vi "Smax.vi"(8 "error in ( error)":errorcluster, 10 "Pair Channel":waveform(sgl), 11 "Data":waveform(sgl)) -> (0 "error out":errorcluster, 3 "Smax":sgl)   [LabVIEW 2017, in "VibrationAnalysisFunctions.lvlib"]
uses:
  <vilib>/addons/InsightCM/Utilities/Analysis/Vibration/VibrationAnalysisFunctions.lvlib
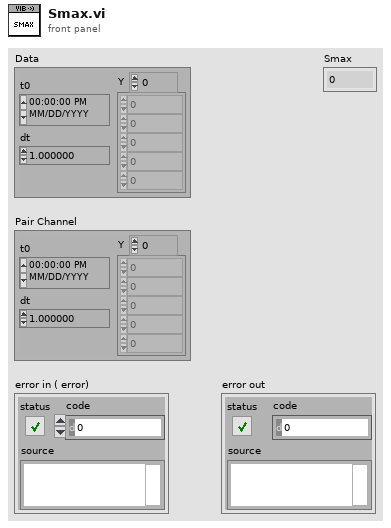
[diagram p1: front panel]
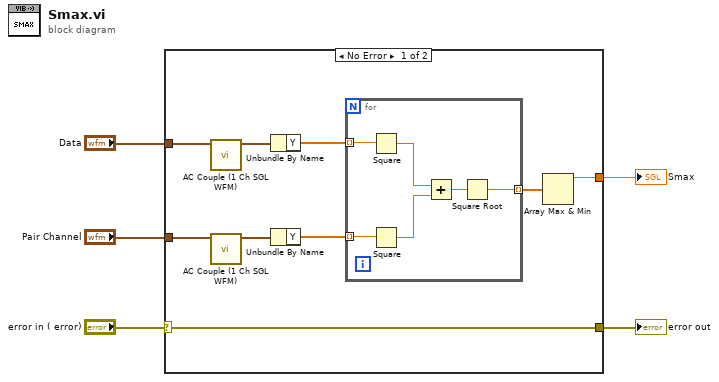
[diagram p0: block diagram]
diagram:
  n1 = case shown="No Error" "error in ( error)" {
    selector: "error in ( error)" -> [w6 w21]
    tunnel: "Data" -> [w12 _]
    tunnel: "Pair Channel" -> [w10 _]
    tunnel: [w7 _] -> w2
    tunnel: [w6 w21] -> w1
    frame No Error {
      n2 = call <vilib>:"AC Couple (1 Ch SGL WFM).vi"("Signal"=w12) -> ("AC Coupled"=w11:waveform(sgl))  [unwired: 8 in, 2 out]
      n3 = call <vilib>:"AC Couple (1 Ch SGL WFM).vi"("Signal"=w10) -> ("AC Coupled"=w9:waveform(sgl))  [unwired: 8 in, 2 out]
      n4 = Unbundle By Name(w11) -> ("Y"=w14:sgl[])
      n5 = Unbundle By Name(w9) -> ("Y"=w13:sgl[])
      n6 = for {
        tunnel: w14 -> [w20] mode=indexing
        tunnel: w13 -> [w19] mode=indexing
        tunnel: [w15] -> w8 mode=indexing
        n7 = Square(x=w20) -> (x^2=w18:sgl)
        n8 = Square(x=w19) -> (x^2=w17:sgl)
        n9 = Add(x=w18, y=w17) -> (x+y=w16:sgl)
        n10 = Square Root(x=w16) -> (sqrt(x)=w15:sgl)
      }
      n11 = Array Max & Min(array=w8) -> (max value=w7:sgl)  [unwired: 3 out]
    }
    frame Error {
    }
  }
  "error out" <- w1
  "Smax" <- w2
